vi "Test Suite Disable Methods.vi"(8 "error in (no error)":errorcluster, 11 "Test Case In":refnum<class "LUnit Test Suite Tests.lvclass">) -> (0 "error out":errorcluster, 3 "Test Case Out":refnum<class "LUnit Test Suite Tests.lvclass">)   [LabVIEW 2020, in "LUnit Test Suite Tests.lvclass"]
uses:
  LUnit Test Suite Tests.lvclass
  C:/Program Files (x86)/National Instruments/LabVIEW 2020/vi.lib/Astemes/LUnit/Test Case.lvclass
  Test Case Test Double Child/Light Test Case Double.lvclass
  C:/Git/astemes-lunit/source/Core/LUnit Test Case/LUnit Test Case.lvclass
  <vilib>/Astemes/LUnit/Test Case.lvclass/Test Case.ctl
  <vilib>/Astemes/LUnit/Palette/Fail.vi
  <vilib>/Astemes/LUnit/Palette/Pass.vi
  <vilib>/Astemes/LUnit/Set Assertion Type.vi
  <vilib>/Astemes/LUnit/Add test result.vi
  <vilib>/Astemes/LUnit/LUnit Record Assertion Result.vi
  <vilib>/Astemes/LUnit/LUnit Aggregate Assertion Results.vi
  <vilib>/Astemes/LUnit/Method Result/LUnit Merge Status.vi
  <vilib>/Astemes/LUnit/LUnit Concatenate result strings.vi
  Mock Result Observer/Mock Result Observer.lvclass
  C:/Git/astemes-lunit/source/Core/Result Observer/Result Observer.lvclass
  Core/LUnit Test Suite/LUnit Test Suite.lvclass
  <vilib>/Astemes/LUnit/Test Case.lvclass
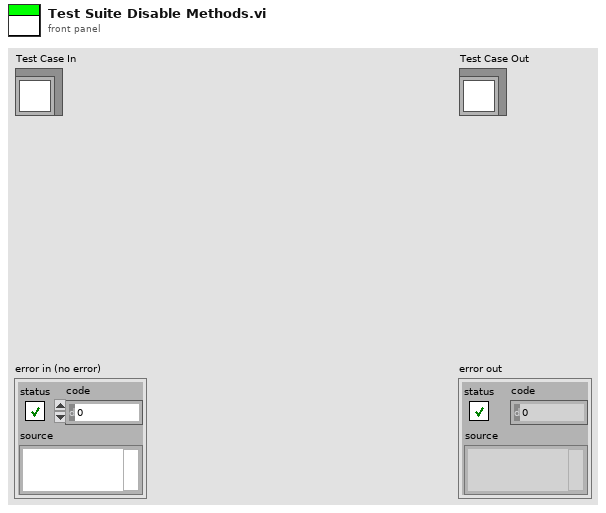
[diagram p1: front panel]
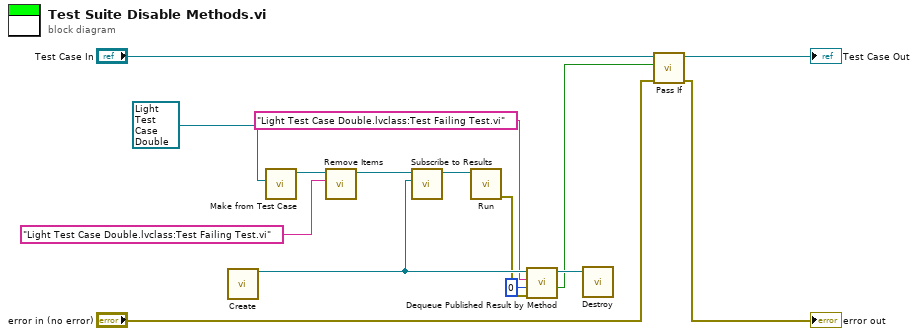
[diagram p0: block diagram]
diagram:
  n1 = call "Create.vi"() -> ("Mock Result Observer out"=w5:refnum<class "Mock Result Observer.lvclass">)  [unwired: 10 in, 1 out]
  n2 = call "Make from Test Case.vi"("LUnit Test Case"=refnum<class "Light Test Case Double.lvclass"> refnum ("Light Test Case Double.lvclass")) -> ("LUnit Test Suite Out"=w11:refnum<class "LUnit Test Suite.lvclass">)  [unwired: 9 in, 1 out]
  n3 = call "Remove Items.vi"("Methods"="Light Test Case Double.lvclass:Test Failing Test.vi", "LUnit Test Suite In"=w11) -> ("LUnit Test Suite Out"=w6:refnum<class "LUnit Test Suite.lvclass">)  [unwired: 8 in, 1 out]
  n4 = call-dynamic "Subscribe to Results.vi"("Result Observer"=w5, "LUnit Test Suite In"=w6) -> ("LUnit Test Suite Out"=w7:refnum<class "LUnit Test Suite.lvclass">)  [unwired: 8 in, 1 out]
  n5 = call-dynamic "Run.vi"("LUnit Test Suite In"=w7) -> ("error out"=w4:errorcluster)  [unwired: 9 in, 1 out]
  n6 = call "Dequeue Published Result by Method.vi"("error in (no error)"=w4, "timeout in ms"=0, "Method Name"="Light Test Case Double.lvclass:Test Failing Test.vi", "Mock Result Observer In"=w5) -> ("timed out?"=w1:bool, "Mock Result Observer Out"=w3:refnum<class "Mock Result Observer.lvclass">)  [unwired: 4 in, 2 out]
  n7 = call "Destroy.vi"("Mock Result Observer in"=w3) -> ()  [unwired: 9 in, 2 out]
  n8 = call <vilib>:"Pass If.vi"("error in (no error)"="error in (no error)", "Pass?"=w1, "LUnit Test Case In"="Test Case In") -> ("error out"=→"error out":errorcluster, "LUnit Test Case Out"=→"Test Case Out":refnum<class "LUnit Test Suite Tests.lvclass">)  [unwired: 7 in]
